vi "main.vi"() -> ()   [LabVIEW 2016, in "Client Controller.lvlib" / "Client Controller.lvclass"]
uses:
  Client Controller.lvclass
  <vilib>/ActorFramework/Message Queue/Message Queue.lvclass/Message Queue.ctl
  <vilib>/ActorFramework/Message Dequeuer/Message Dequeuer.lvclass/Message Dequeuer.ctl
  C:/Program Files (x86)/National Instruments/LabVIEW 2016/vi.lib/ActorFramework/Actor/Actor.lvclass
  <vilib>/ActorFramework/Message Priority Queue/Priority Dequeue.vi
  <vilib>/ActorFramework/Actor/Actor.lvclass
  <vilib>/ActorFramework/Message Queue/Message Queue.lvclass
  <vilib>/ActorFramework/Message Dequeuer/Message Dequeuer.lvclass
  MAL-Framework/user.lib/Common Components/Controller/Controller.lvclass
panel:
  out "String":string
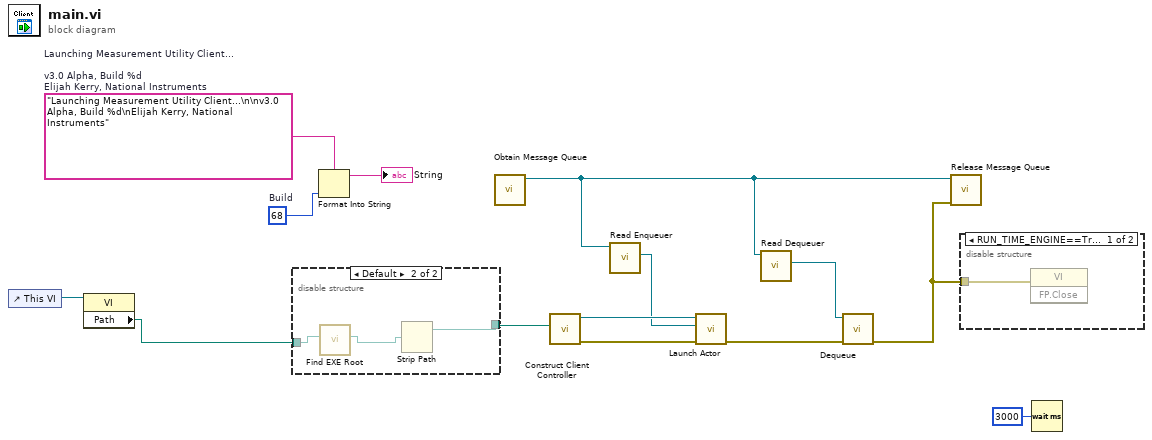
[diagram p0: block diagram]
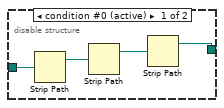
[diagram p2: hidden frame]
diagram:
  w3 = 68  # Build
  w5 = "Launching Measurement Utility Client...\n\nv3.0 Alpha, Build %d\nElijah Kerry, National Instruments"  # Launching Measurement Utility Client...  v3.0 Alpha, Build %d Elijah Kerry, National Instruments
  n1 = control-ref of="This VI"() -> (w12:refnum<vi>)
  n2 = property class="VI"(reference=w12) -> ("Path"=w1:path)  [unwired: 1 in, 2 out]
  n3 = disable-structure shown="Default" {
    disable-tunnel: w1 -> [w17 w20]
    disable-tunnel: [w15 w21] -> w2
    frame condition #0 (active) {
      n4 = Strip Path(path=w17) -> (stripped path=w18:path)  [unwired: 1 out]
      n5 = Strip Path(path=w18) -> (stripped path=w16:path)  [unwired: 1 out]
      n6 = Strip Path(path=w16) -> (stripped path=w15:path)  [unwired: 1 out]
    }
    frame condition #1 {
      n7 = call "Find EXE Root.vi"("Path"=w20) -> ("Location of EXE"=w19:path)  [unwired: 10 in]
      n8 = Strip Path(path=w19) -> (stripped path=w21:path)  [unwired: 1 out]
    }
  }
  n9 = Format Into String(format string=w5, w3) -> (resulting string=→"String":string)  [unwired: 2 in, 1 out]
  n10 = call <vilib>:"Obtain Message Queue.vi"() -> ("Message Queue"=w10:refnum<class "Message Queue.lvclass">)  [unwired: 10 in, 1 out]
  n11 = call "Construct Client Controller.vi"("Base Path"=w2) -> ("error out"=w13:errorcluster, "Client Controller out"=w14:refnum<class "Client Controller.lvclass">)  [unwired: 9 in]
  n12 = call <vilib>:"Read Enqueuer.vi"("Message Queue"=w10) -> ("Message Enqueuer"=w11:refnum<class "Message Enqueuer.lvclass">)  [unwired: 10 in]
  n13 = call <vilib>:"Launch Actor.vi"("error in (no error)"=w13, "Actor-to-Caller Enqueuer"=w11, "Actor"=w14) -> ("error out"=w9:errorcluster)  [unwired: 7 in, 1 out]
  n14 = call <vilib>:"Read Dequeuer.vi"("Message Queue"=w10) -> ("Message Dequeuer"=w8:refnum<class "Message Dequeuer.lvclass">)  [unwired: 10 in]
  n15 = call <vilib>:"Dequeue.vi"("error in (no error)"=w9, "Message Dequeuer in"=w8) -> ("error out"=w7:errorcluster)  [unwired: 5 in, 4 out]
  n16 = call <vilib>:"Release Message Queue.vi"("error in (no error)"=w7, "Message Queue"=w10) -> ()  [unwired: 8 in, 2 out]
  n17 = disable-structure shown="RUN_TIME_ENGINE==True" {
    disable-tunnel: w7 -> [w22 _]
    frame condition #0 {
      n18 = invoke class="VI" method="FP.Close"(error in=w22) -> ()  [unwired: 2 in, 3 out]
    }
    frame condition #1 (active) {
    }
  }
  n19 = Wait (ms)(milliseconds to wait=u32 3000) -> ()  [unwired: 1 out]
